vi "test Get Set Analog Replay.vi"(8 "error in (no error)":errorcluster, 11 "TestCase in":refnum<class "Scripting API Test Case.lvclass">) -> (0 "error out":errorcluster, 3 "TestCase out":refnum<class "Scripting API Test Case.lvclass">)   [LabVIEW 2020, in "Scripting API Test Case.lvclass"]
uses:
  Scripting API Test Case.lvclass
  Scripting API/Custom Device/Engine Simulation Toolkit Custom Device Settings.ctl
  Scripting API/Bitfile/Bitfile.ctl
  Scripting API/Analog Replay/Analog Replay Settings.ctl
  Scripting API/Analog Replay/Analog Replay Data Options.ctl
  System Explorer/FPGA Mem Size.ctl
  System Explorer/Position Reference.ctl
  System Explorer/Data Replay Data Selection Method.ctl
  Scripting API Test Case.lvclass/Scripting API Test Case.ctl
  <userlib>/_OpenG.lib/file/file.llb/Append Path to Root if Relative - Scalar__ogtk.vi
  <vilib>/addons/_JKI Toolkits/VI Tester/TestCase.llb/TestCase.lvclass
  <vilib>/NI/VeriStand Custom Device Testing Tools/VeriStandTestUtilities/VeriStandTestUtilities.lvlib
  Scripting API/Engine Simulation Toolkit Scripting API.lvlib
  System Explorer/Engine Simulation Toolkit System Explorer.lvlib
  C:/Program Files (x86)/National Instruments/LabVIEW 2020/vi.lib/addons/_JKI Toolkits/VI Tester/TestCase.llb/TestCase.lvclass
panel:
  in  "Save?":bool
  out "Output Filename":string
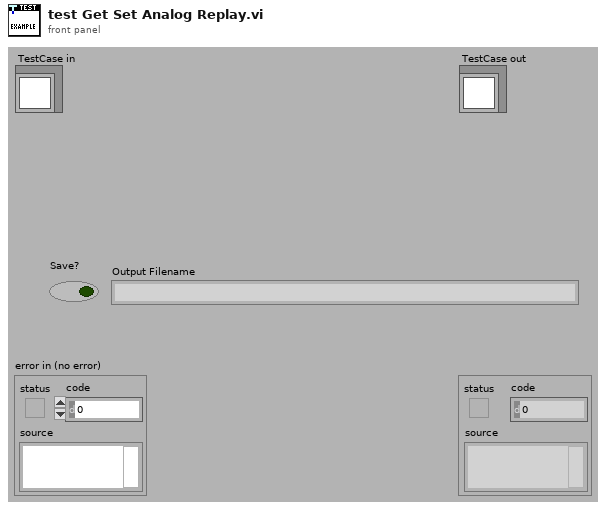
[diagram p1: front panel]
types:
  T1 = typedef "Engine Simulation Toolkit Scripting API.lvlib/Analog Replay Data Options.ctl" = cluster{"Selected File":path, "Group":string, "Channel":string, "DataPlugin":string, "ReverseData":bool, "FPGA memory size":T2, "CycleAngle?":T3, "Data Selection Method":T4, "File start offset":i32, "Samples":i32, "Missing teeth location (degrees)":dbl}
  T2 = typedef "Engine Simulation Toolkit System Explorer.lvlib/FPGA Mem Size.ctl" = enum16{"65,536", "32,768", "16,384", "8,192", "4,096", "2,048", "1,024"}
  T3 = typedef "Engine Simulation Toolkit System Explorer.lvlib/Position Reference.ctl" = enum16{"Crank angle", "Cycle angle"}
  T4 = typedef "Engine Simulation Toolkit System Explorer.lvlib/Data Replay Data Selection Method.ctl" = enum32{"Manual", "AutoVRCrank"}
  T5 = typedef "Engine Simulation Toolkit Scripting API.lvlib/Bitfile.ctl" = cluster{"RIO Device Address":string, "Bitfile Path":path}
  T6 = typedef "Engine Simulation Toolkit Scripting API.lvlib/Engine Simulation Toolkit Custom Device Settings.ctl" = cluster{"Name":string, "Execution priority":enum16{"Low", "Medium", "High"}, "Rate decimation":i32, "CPU":i32}
  T7 = typedef "Engine Simulation Toolkit Scripting API.lvlib/Analog Replay Settings.ctl" = cluster{"Name":string, "RIO Device Address":string, "DAC bipolar range (V)":dbl, "Voltage below min speed":dbl, "Min speed (RPM)":dbl, "Voltage at min speed":dbl, "Max speed (RPM)":dbl, "Voltage at max speed":dbl, "ReverseNegate":bool, "VOverride":bool}
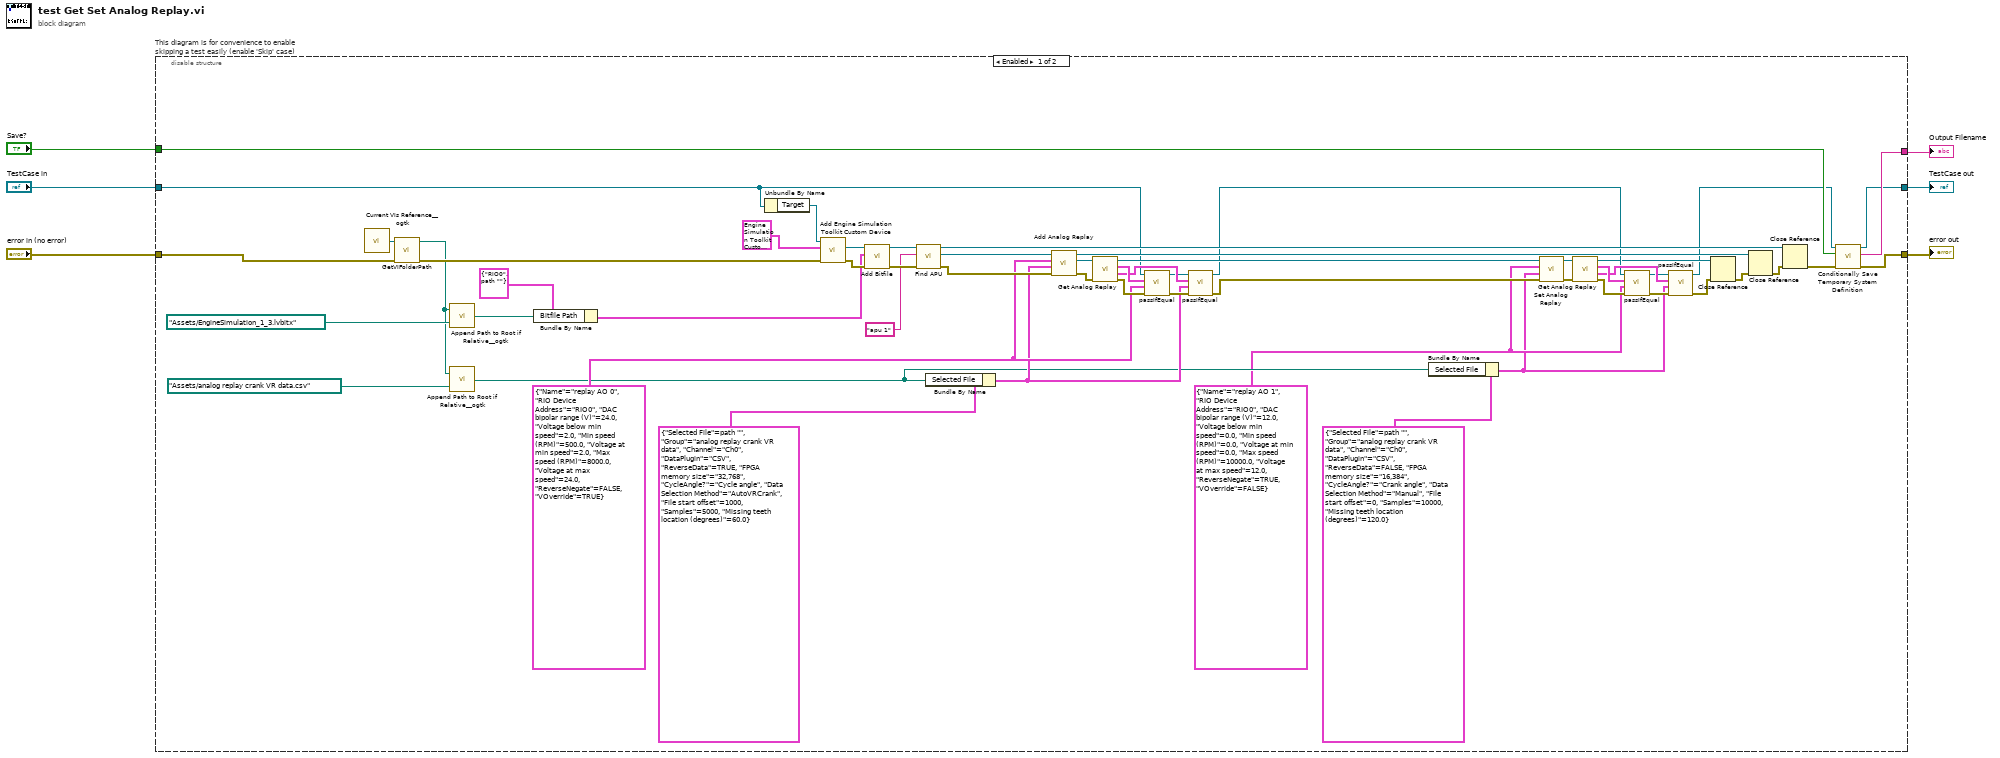
[diagram p0: block diagram]
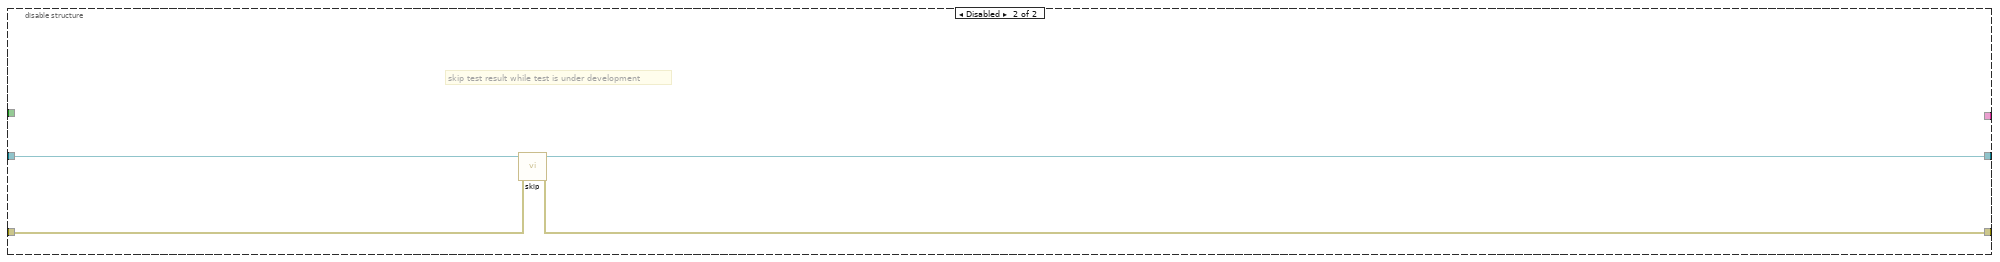
[diagram p2: hidden frame]
diagram:
  n1 = disable-structure "This diagram is for convenience to enable skipping a test easily (enable 'Skip' case)" shown="Enabled" {
    disable-tunnel: "TestCase in" -> [w8 w65]
    disable-tunnel: [w9 w63] -> w3
    disable-tunnel: [w57 w64] -> w5
    disable-tunnel: "error in (no error)" -> [w60 w62]
    disable-tunnel: [w56 _] -> w2
    disable-tunnel: "Save?" -> [w55 _]
    frame Enabled {
      w15 = T7 {"Name"="replay AO 1", "RIO Device Address"="RIO0", "DAC bipolar range (V)"=12.0, "Voltage below min speed"=0.0, "Min speed (RPM)"=0.0, "Voltage at min speed"=0.0, "Max speed (RPM)"=10000.0, "Voltage at max speed"=12.0, "ReverseNegate"=TRUE, "VOverride"=FALSE} ("Analog Replay Settings")
      w31 = T7 {"Name"="replay AO 0", "RIO Device Address"="RIO0", "DAC bipolar range (V)"=24.0, "Voltage below min speed"=2.0, "Min speed (RPM)"=500.0, "Voltage at min speed"=2.0, "Max speed (RPM)"=8000.0, "Voltage at max speed"=24.0, "ReverseNegate"=FALSE, "VOverride"=TRUE} ("Analog Replay Settings")
      n2 = call <userlib>:"Current VIs Reference__ogtk.vi"() -> ("Current VI's reference"=w61:refnum<vi>)  [unwired: 5 in]
      n3 = call <vilib>:"GetVIFolderPath.vi"("error in (no error)"=w60, "VI Reference in"=w61) -> ("error out"=w59:errorcluster, "VI Folder Path out"=w41:path)  [unwired: 8 in]
      n4 = call-poly <userlib>:"Append Path to Root if Relative__ogtk.vi"("Absolute or Relative Path"=path "Assets/EngineSimulation_1_3.lvbitx", "Root Path"=w41) -> ("Absolute or Appended Path"=w48:path)
      n5 = call-poly <userlib>:"Append Path to Root if Relative__ogtk.vi"("Absolute or Relative Path"=path "Assets/analog replay crank VR data.csv", "Root Path"=w41) -> ("Absolute or Appended Path"=w24:path)
      n6 = Bundle By Name(cluster=T5 {"RIO Device Address"="RIO0", "Bitfile Path"=path ""} ("Engine Simulation Toolkit Bitfile"), "Bitfile Path"=w48) -> (w49:T5)
      n7 = Unbundle By Name(w8) -> ("Target"=w7:refnum<k24>)
      n8 = call "Add Engine Simulation Toolkit Custom Device.vi"("error in (no error)"=w59, "Settings"=T6 {"Name"="Engine Simulation Toolkit Custom Device", "Execution priority"=enum."Medium", "Rate decimation"=1, "CPU"=-2} ("Engine Simulation Toolkit Custom Device Settings"), "Target in"=w7) -> ("error out"=w52:errorcluster, "EST Custom Device"=w54:refnum<k24>)  [unwired: 6 in, 1 out]
      n9 = call "Add Bitfile.vi"("error in (no error)"=w52, "Engine Simulation Toolkit Bitfile"=w49, "EST Custom Device in"=w54) -> ("error out"=w46:errorcluster, "EST Custom Device out"=w47:refnum<k24>)  [unwired: 7 in]
      n10 = call "Find APU.vi"("error in (no error)"=w46, "Name"="apu 1", "EST Custom Device in"=w47) -> ("error out"=w38:errorcluster, "APU"=w39:refnum<k24>, "EST Custom Device out"=w45:refnum<k24>)  [unwired: 6 in]
      n11 = Bundle By Name(cluster=T1 {"Selected File"=path "", "Group"="analog replay crank VR data", "Channel"="Ch0", "DataPlugin"="CSV", "ReverseData"=TRUE, "FPGA memory size"=enum."32,768", "CycleAngle?"=enum."Cycle angle", "Data Selection Method"=enum."AutoVRCrank", "File start offset"=1000, "Samples"=5000, "Missing teeth location (degrees)"=60.0} ("Analog Replay Data Options"), "Selected File"=w24) -> (w29:T1)
      n12 = call "Add Analog Replay.vi"("error in (no error)"=w38, "Analog Replay Data Options"=w29, "Analog Replay Settings"=w31, "APU in"=w39) -> ("error out"=w37:errorcluster, "Analog Replay"=w36:refnum<k24>, "APU out"=w27:refnum<k24>)  [unwired: 5 in]
      n13 = call "Get Analog Replay.vi"("error in (no error)"=w37, "Analog Replay in"=w36) -> ("error out"=w35:errorcluster, "Analog Replay Data Options"=w30:T1, "Analog Replay Settings"=w32:T7, "Analog Replay out"=w28:refnum<k24>)  [unwired: 6 in]
      n14 = call-dynamic "passIfEqual.vi"("error in (no error)"=w35, "y"=w31, "x"=w32, "TestCase in"=w8) -> ("error out"=w33:errorcluster, "TestCase out"=w26:refnum<class "Scripting API Test Case.lvclass">)  [unwired: 6 in]
      n15 = call-dynamic "passIfEqual.vi"("error in (no error)"=w33, "y"=w29, "x"=w30, "TestCase in"=w26) -> ("error out"=w34:errorcluster, "TestCase out"=w16:refnum<class "Scripting API Test Case.lvclass">)  [unwired: 6 in]
      n16 = Bundle By Name(cluster=T1 {"Selected File"=path "", "Group"="analog replay crank VR data", "Channel"="Ch0", "DataPlugin"="CSV", "ReverseData"=FALSE, "FPGA memory size"=enum."16,384", "CycleAngle?"=enum."Crank angle", "Data Selection Method"=enum."Manual", "File start offset"=0, "Samples"=10000, "Missing teeth location (degrees)"=120.0} ("Analog Replay Data Options"), "Selected File"=w24) -> (w14:T1)
      n17 = call "Set Analog Replay.vi"("error in (no error)"=w34, "Analog Replay Data Options"=w14, "Analog Replay Settings"=w15, "Analog Replay in"=w28) -> ("error out"=w17:errorcluster, "Analog Replay out"=w18:refnum<k24>)  [unwired: 6 in]
      n18 = call "Get Analog Replay.vi"("error in (no error)"=w17, "Analog Replay in"=w18) -> ("error out"=w23:errorcluster, "Analog Replay Data Options"=w20:T1, "Analog Replay Settings"=w21:T7, "Analog Replay out"=w11:refnum<k24>)  [unwired: 6 in]
      n19 = call-dynamic "passIfEqual.vi"("error in (no error)"=w23, "y"=w15, "x"=w21, "TestCase in"=w16) -> ("error out"=w22:errorcluster, "TestCase out"=w19:refnum<class "Scripting API Test Case.lvclass">)  [unwired: 6 in]
      n20 = call-dynamic "passIfEqual.vi"("error in (no error)"=w22, "y"=w14, "x"=w20, "TestCase in"=w19) -> ("error out"=w12:errorcluster, "TestCase out"=w10:refnum<class "Scripting API Test Case.lvclass">)  [unwired: 6 in]
      n21 = Close Reference(reference=w11, error in (no error)=w12) -> (error out=w13:errorcluster)
      n22 = Close Reference(reference=w27, error in (no error)=w13) -> (error out=w43:errorcluster)
      n23 = Close Reference(reference=w45, error in (no error)=w43) -> (error out=w58:errorcluster)
      n24 = call "Conditionally Save Temporary System Definition.vi"("error in (no error)"=w58, "Save?"=w55, "Test Case"=w10) -> ("error out"=w57:errorcluster, "filename"=w56:string, "Test Case"=w9:refnum<class "Scripting API Test Case.lvclass">)  [unwired: 6 in]
    }
    frame Disabled {
      # "skip test result while test is under development"
      n25 = call <vilib>:"skip.vi"("error in (no error)"=w62, "TestCase in"=w65) -> ("error out"=w64:errorcluster, "TestCase out"=w63:refnum<class "Scripting API Test Case.lvclass">)  [unwired: 8 in]
    }
  }
  "error out" <- w5
  "TestCase out" <- w3
  "Output Filename" <- w2
